vi "subSave_CreateSubfolder.vi"(7 "Time (F)":bool, 8 "Subfolder name":string="MC3D_", 11 "Base path":path=path "C:/Peng/Data/20160201 test") -> (3 "Subfolder":path=path "C:/Peng/Data/20160201 test/172659_MC3D_")   [LabVIEW 2015]
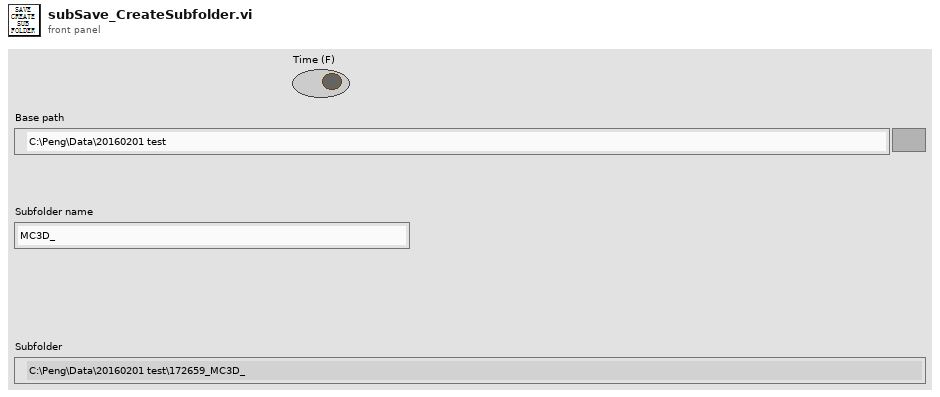
[diagram p1: front panel]
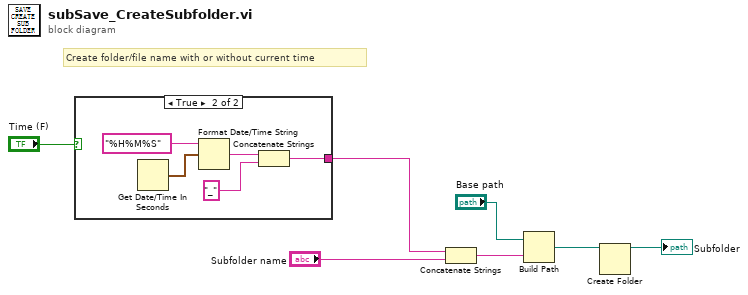
[diagram p0: block diagram]
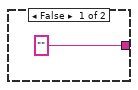
[diagram p2: hidden frame]
diagram:
  # "Create folder/file name with or without current time"
  n1 = case shown="True" "Time (F)" {
    tunnel: ["" w9] -> w6
    frame False {
    }
    frame True {
      n2 = Get Date/Time In Seconds() -> (seconds since 1Jan1904=w12:timestamp)
      n3 = Format Date/Time String(time format string (%c)="%H%M%S", seconds (now)=w12) -> (date/time string=w11:string)  [unwired: 1 in]
      n4 = Concatenate Strings(w11, "_") -> (w9:string)
    }
  }
  n5 = Concatenate Strings(w6, "Subfolder name") -> (w3:string)
  n6 = Build Path(base path="Base path", name or relative path=w3) -> (appended path=w4:path)
  n7 = Create Folder(path (use dialog)=w4) -> (created path=→"Subfolder":path)  [unwired: 2 in, 2 out]
